vi "Handle Notification.vi"(8 "error in (no error)":errorcluster, 9 "Payload":string, 10 "Notification Type":string, 11 "Test Sequencer in":refnum<class "Output Sequencer.lvclass">) -> (0 "error out":errorcluster, 3 "Test Sequencer out":refnum<class "Output Sequencer.lvclass">)   [LabVIEW 2020, in "Output Sequencer.lvlib" / "Output Sequencer.lvclass"]
uses:
  Output Sequencer.lvclass
  Output Sequencer.lvclass/Output Sequencer.ctl
  Types/Sequencer State.ctl
  Types/Event Type.ctl
  Types/UI Event.ctl
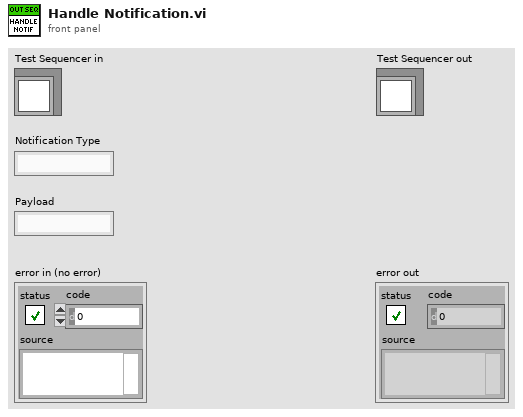
[diagram p1: front panel]
types:
  T1 = typedef "Output Sequencer.lvlib/Output Sequencer.lvclass/UI Ref.ctl" = refnum<vi>
  T2 = typedef "Output Sequencer.lvlib/Output Sequencer.lvclass/Sequencer State.ctl" = enum16{"Error", "Initialize", "Prepare channels", "Wait for test", "Wait for %.1f sec", "Wait for trigger", "Stop condition", "Wait for resume", "Running", "Paused", "No valid step", "Stopped"}
  T3 = typedef "Output Sequencer.lvlib/Output Sequencer.lvclass/Event Type.ctl" = enum16{"Channel Update", "Test State Change", "Stop"}
  T4 = typedef "Output Sequencer.lvlib/Output Sequencer.lvclass/UI Event.ctl" = cluster{"Type":T3, "Data":variant}
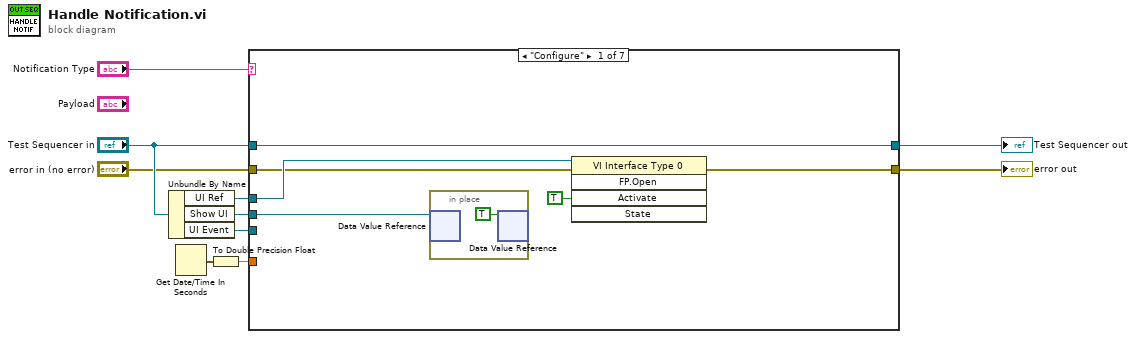
[diagram p0: block diagram]
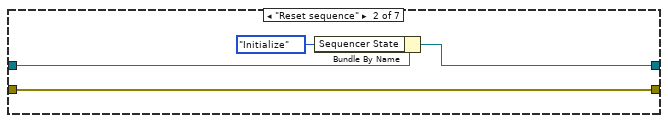
[diagram p2: hidden frame]
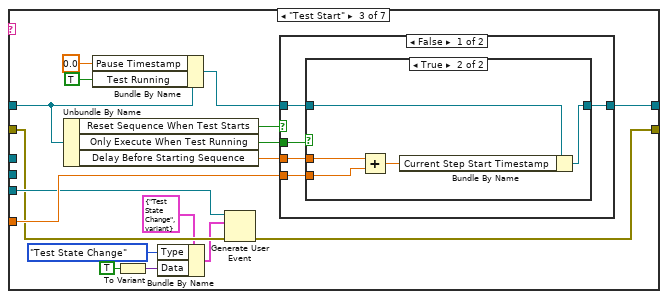
[diagram p3: hidden frame]
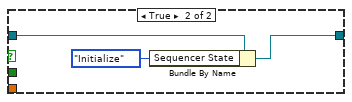
[diagram p5: hidden frame]
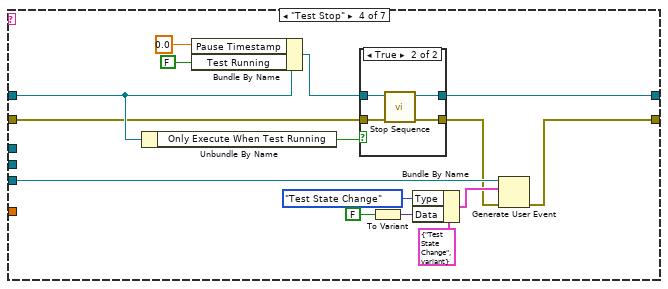
[diagram p6: hidden frame]
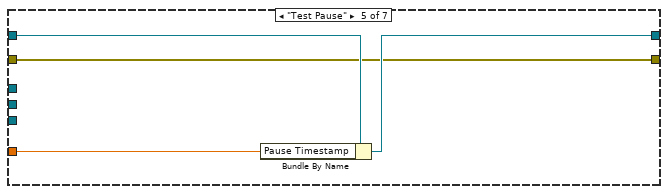
[diagram p8: hidden frame]
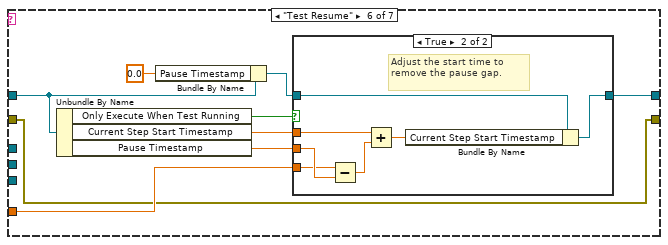
[diagram p9: hidden frame]
diagram:
  n1 = Unbundle By Name("Test Sequencer in") -> ("UI Ref"=w7:T1, "Show UI"=w6:refnum<data-value>, "UI Event"=w3:refnum<user-event>)
  n2 = Get Date/Time In Seconds() -> (seconds since 1Jan1904=w9:timestamp)
  n3 = To Double Precision Float(number=w9) -> (double precision float=w8:dbl)
  n4 = case shown="\"Configure\"" "Notification Type" {
    tunnel: "Test Sequencer in" -> [w15 w20 w38 w67 w75 w86 w96]
    tunnel: [w15 w21 w37 w64 w77 w84 w96] -> w4
    tunnel: w8 -> [_ _ w36 _ w76 w79 _]
    tunnel: w7 -> [w16 _ _ _ _ _ _]
    tunnel: w6 -> [w14 _ _ _ _ _ _]
    tunnel: w3 -> [_ _ w35 w56 _ _ _]
    tunnel: "error in (no error)" -> [w13 w19 w34 w55 w74 w78 w95]
    tunnel: [w12 w19 w33 w53 w74 w78 w95] -> w1
    frame "Configure" {
      n5 = in-place {
        n6 = in-place-dvr #1(w14) -> ()  [unwired: 2 out]
        n7 = in-place-dvr #1(TRUE ("data value")) -> ()  [unwired: 2 out]
      }
      n8 = invoke class="VI Interface Type 0" method="FP.Open"(reference=w16, error in=w13, "Activate"=TRUE ("Activate?")) -> (error out=w12:errorcluster)  [unwired: 2 in, 4 out]
    }
    frame "Reset sequence" {
      n9 = Bundle By Name(cluster=w20, "Sequencer State"=Sequencer_State."Initialize" ("State.Sequencer State")) -> (w21:refnum<class "Output Sequencer.lvclass">)
    }
    frame "Test Start" {
      n10 = Unbundle By Name(w38) -> ("Reset Sequence When Test Starts"=w28:bool, "Only Execute When Test Running"=w27:bool, "Delay Before Starting Sequence"=w29:dbl)
      n11 = Bundle By Name(cluster=w38, "Pause Timestamp"=0.0, "Test Running"=TRUE) -> (w31:refnum<class "Output Sequencer.lvclass">)
      n12 = To Variant(anything=TRUE ("Test In Progress")) -> (Variant=w24:variant)
      n13 = Bundle By Name(cluster=T4 {"Type"=enum."Test State Change", "Data"=variant} ("UI Event"), "Type"=Event_Type."Test State Change", "Data"=w24) -> (w26:T4)
      n14 = Generate User Event(user event=w35, event data cluster=w26, error in=w34) -> (error out=w33:errorcluster)  [unwired: 1 in, 1 out]
      n15 = case shown="False" w28 {
        tunnel: w31 -> [w43 w52]
        tunnel: [w42 w51] -> w37
        tunnel: w36 -> [w41 _]
        tunnel: w29 -> [w40 _]
        tunnel: w27 -> [w39 _]
        frame False {
          n16 = case shown="True" w39 {
            tunnel: [w44 w49] -> w42
            tunnel: w43 -> [w44 w48]
            tunnel: w41 -> [_ w47]
            tunnel: w40 -> [_ w46]
            frame False {
            }
            frame True {
              n17 = Add(x=w46, y=w47) -> (x+y=w45:dbl)
              n18 = Bundle By Name(cluster=w48, "Current Step Start Timestamp"=w45) -> (w49:refnum<class "Output Sequencer.lvclass">)
            }
          }
        }
        frame True {
          n19 = Bundle By Name(cluster=w52, "Sequencer State"=Sequencer_State."Initialize" ("State.Sequencer State")) -> (w51:refnum<class "Output Sequencer.lvclass">)
        }
      }
    }
    frame "Test Stop" {
      n20 = Unbundle By Name(w67) -> ("Only Execute When Test Running"=w66:bool)
      n21 = Bundle By Name(cluster=w67, "Pause Timestamp"=0.0, "Test Running"=FALSE) -> (w65:refnum<class "Output Sequencer.lvclass">)
      n22 = case shown="True" w66 {
        tunnel: w65 -> [w69 w73]
        tunnel: [w69 w72] -> w64
        tunnel: w55 -> [w68 w71]
        tunnel: [w68 w70] -> w54
        frame False {
        }
        frame True {
          n23 = call "Stop Sequence.vi"("error in (no error)"=w71, "Output Sequencer in"=w73) -> ("error out"=w70:errorcluster, "Output Sequencer out"=w72:refnum<class "Output Sequencer.lvclass">)  [unwired: 7 in, 1 out]
        }
      }
      n24 = To Variant(anything=FALSE ("Test In Progress")) -> (Variant=w60:variant)
      n25 = Bundle By Name(cluster=T4 {"Type"=enum."Test State Change", "Data"=variant} ("UI Event"), "Type"=Event_Type."Test State Change", "Data"=w60) -> (w61:T4)
      n26 = Generate User Event(user event=w56, event data cluster=w61, error in=w54) -> (error out=w53:errorcluster)  [unwired: 1 in, 1 out]
    }
    frame "Test Pause" {
      n27 = Bundle By Name(cluster=w75, "Pause Timestamp"=w76) -> (w77:refnum<class "Output Sequencer.lvclass">)
    }
    frame "Test Resume" {
      n28 = Unbundle By Name(w86) -> ("Only Execute When Test Running"=w83:bool, "Current Step Start Timestamp"=w81:dbl, "Pause Timestamp"=w80:dbl)
      n29 = Bundle By Name(cluster=w86, "Pause Timestamp"=0.0) -> (w85:refnum<class "Output Sequencer.lvclass">)
      n30 = case shown="True" w83 {
        tunnel: w85 -> [w87 w94]
        tunnel: [w87 w93] -> w84
        tunnel: w81 -> [_ w91]
        tunnel: w80 -> [_ w90]
        tunnel: w79 -> [_ w89]
        frame False {
        }
        frame True {
          # "Adjust the start time to remove the pause gap."
          n31 = Subtract(x=w89, y=w90) -> (x-y=w92:dbl)
          n32 = Add(x=w91, y=w92) -> (x+y=w88:dbl)
          n33 = Bundle By Name(cluster=w94, "Current Step Start Timestamp"=w88) -> (w93:refnum<class "Output Sequencer.lvclass">)
        }
      }
    }
    frame Default {
    }
  }
  "error out" <- w1
  "Test Sequencer out" <- w4
